vi "picADC graph.vi"() -> ()   [LabVIEW 2014]
doc: "This example performs a serial port write and a serial port read. The parameters set for the serial port must match the parameters of the connected instrument or device. The VISA Configure Serial Port VI sets the configuration parameters. The front panel displays the controls used to configure the basic parameters, such as baud rate, data bits, and parity. The VI passes the VISA resource name to other VIs that perform operations on that VISA resource. The VISA Write function sends a command to the serial device and the VISA Read function returns data based on the command. The VISA Close function then closes the reference to the serial device. It is important to close the reference; otherwise, further communication through that port might not be possible."
uses:
  Program Files (x86)/National Instruments/LabVIEW 2014/examples/Instrument IO/Serial/support/Serial - Settings.ctl
  <vilib>/Instr/_visa.llb/VISA Configure Serial Port (Instr).vi
panel:
  out "byte array":u8[](array[numeric]) format="%02x"
  out "Waveform":u16(graph)
  in  "stop":bool
  in  "Serial Settings":T1={"baud rate"=115200, "data bits"=8, "parity"=enum."None", "stop bits"=10, "flow control"=0} {"flow control" items=["None"=0, "XON/XOFF"=1, "RTS/CTS"=2, "DTR/DSR"=4]; "stop bits" items=["1.0"=10, "1.5"=15, "2.0"=20]; "data bits" min=5 max=8 step=1; "baud rate" items=["75"=75, "110"=110, "134"=134, "150"=150, "300"=300, "600"=600, "1200"=1200, "1800"=1800, "2400"=2400, "4800"=4800, "7200"=7200, "9600"=9600, "14400"=14400, "19200"=19200, "28800"=28800, "38400"=38400, "56000"=56000, "57600"=57600, "115200"=115200, "128000"=128000, "230400"=230400]}
  in  "VISA resource name":refnum<visa-resource-name>="COM2"
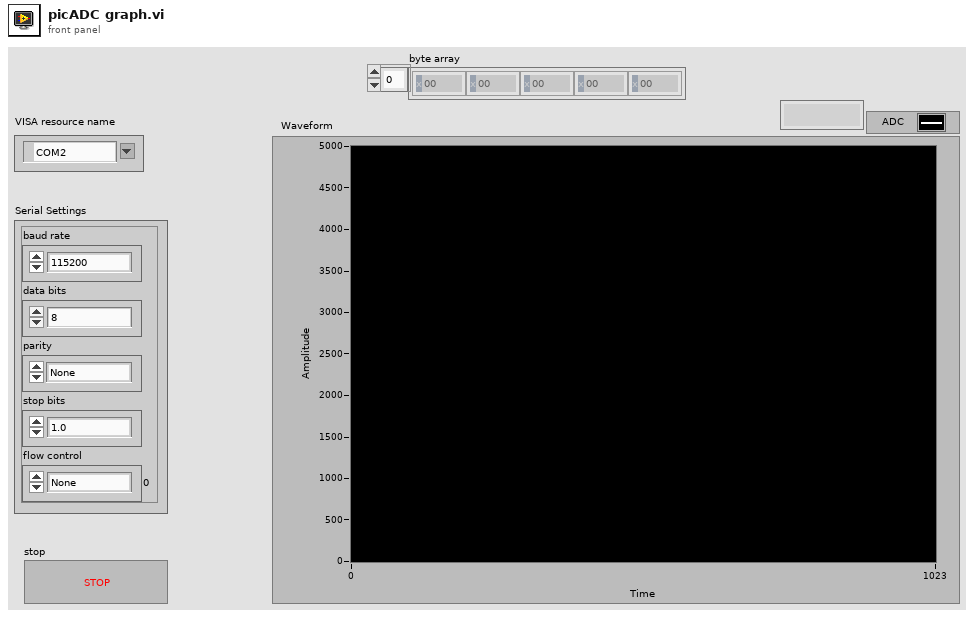
[diagram p1: front panel]
types:
  T1 = typedef "Serial - Settings.ctl" = cluster{"baud rate":u32, "data bits":u16, "parity":enum16{"None", "Odd", "Even", "Mark", "Space"}, "stop bits":u16, "flow control":u16}
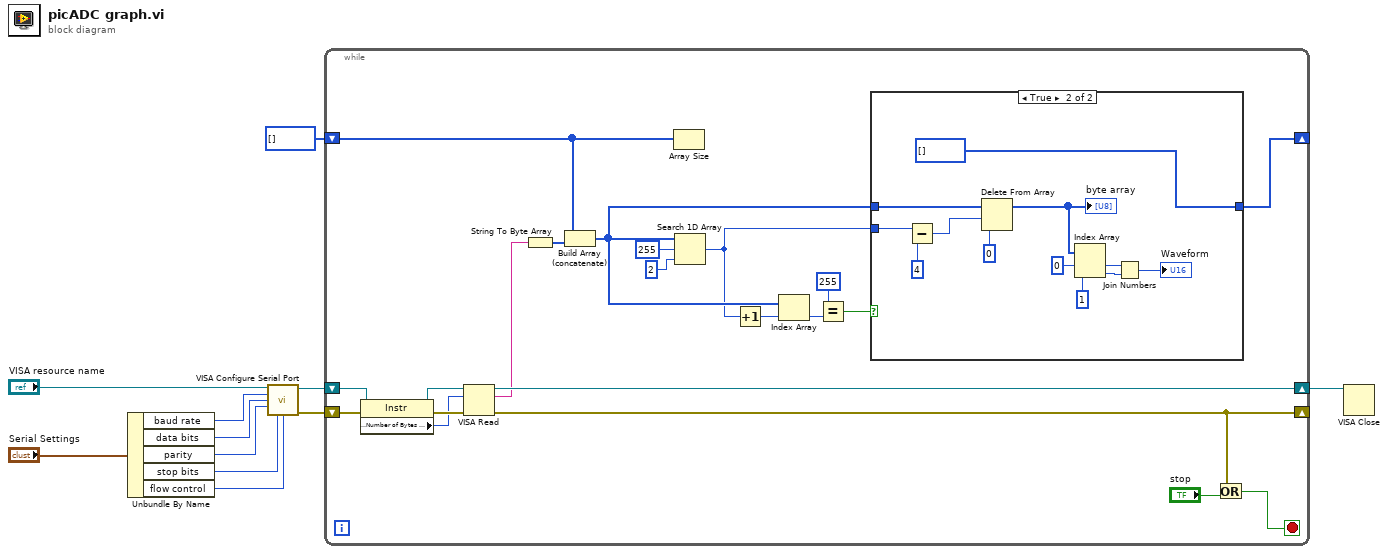
[diagram p0: block diagram]
diagram:
  n1 = Unbundle By Name("Serial Settings") -> ("baud rate"=w8:u32, "data bits"=w7:u16, "parity"=w6:enum16{"None", "Odd", "Even", "Mark", "Space"}, "stop bits"=w5:u16, "flow control"=w4:u16)
  n2 = call-poly "VISA Configure Serial Port"("VISA resource name"="VISA resource name", "baud rate (9600)"=w8, "data bits (8)"=w7, "parity (0:none)"=w6, "stop bits (10: 1 bit)"=w5, "flow control (0:none)"=w4) -> ("VISA resource name out"=w2:refnum<visa-resource-name>, "error out"=w3:errorcluster)  [unwired: 3 in, 5 out]
  n3 = while {
    shift-right: [w30] -> _
    shift-left: w3 -> [w26]
    shift-right: [w32] -> w10
    shift-left: w2 -> [w28]
    shift-right: [w19] -> _
    shift-left: u8[] [] -> [w18]
    stop <- w22 stop-if-true
    n4 = property class="Instr"(reference=w28, error in=w26) -> (reference out=w27:refnum<visa-resource-name>, error out=w25:errorcluster, "Serial Settings:Number of Bytes at Serial Port"=w24:u32)
    n5 = VISA Read(VISA resource name=w27, byte count=w24, error in (no error)=w25) -> (VISA resource name out=w32:refnum<visa-resource-name>, read buffer=w31:string, error out=w30:errorcluster)  [unwired: 1 out]
    n6 = String To Byte Array(string=w31) -> (unsigned byte array=w21:u8[])
    n7 = Build Array (concatenate)(w18, w21) -> (w16:u8[])
    n8 = Array Size(array=w18) -> ()  [unwired: 1 out]
    n9 = Search 1D Array(1D array=w16, element=u8 255, start index (0)=2) -> (index of element=w13:i32)
    n10 = Increment(x=w13) -> (x+1=w12:i32)
    n11 = Index Array(array=w16, index=w12) -> (element=w15:u8)
    n12 = Equal?(x=u8 255 ("element"), y=w15) -> (x = y?=w20:bool)
    n13 = case shown="True" w20 {
      tunnel: w16 -> [w33 w39]
      tunnel: [w33 u8[] []] -> w19
      tunnel: w13 -> [_ w35]
      frame False {
      }
      frame True {
        n14 = Subtract(x=w35, y=4) -> (x-y=w36:i32)
        n15 = Delete From Array(array=w39, length=w36, index=0) -> (array with subset deleted=w37:u8[])  [unwired: 1 out]
        "byte array" <- w37
        n16 = Index Array(array=w37, index #1=0 ("index"), index #2=1 ("index")) -> (element #1=w43:u8, element #2=w44:u8)
        n17 = Join Numbers(hi=w43, lo=w44) -> ((hi.lo)=→"Waveform":u16)
      }
    }
    n18 = Or(x=w30, y="stop") -> (x .or. y?=w22:bool)
  }
  n19 = VISA Close(VISA resource name=w10) -> ()  [unwired: 1 in, 1 out]
